vi "Rodriguez_Ex3Task1_Main.vi"() -> ()   [LabVIEW 2014, in "Rodriguez1_Visage_5th_LegoRobotics_11-29-16.lvrbt"]
uses:
  Rodriguez1_Visage_5th_LegoRobotics_11-29-16.lvrbt
panel:
  out "Current Distance":dbl
  in  "Max Distance":dbl
  in  "Min Distance":dbl
  out "Wall Proximity":string
  out "Distance LED":bool
  in  "stop":bool
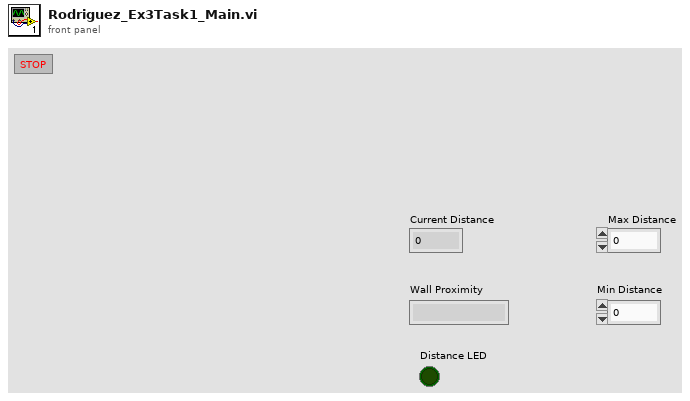
[diagram p1: front panel]
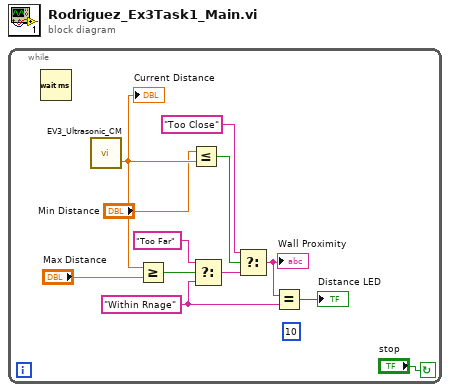
[diagram p0: block diagram]
diagram:
  n1 = while {
    stop <- "stop" continue-if-true
    (unwired) u32 10 ("millisecond timer value")
    w4 = "Within Rnage"
    n2 = Wait (ms)() -> ()  [unwired: 1 in, 1 out]
    n3 = call <vilib>:"EV3_Ultrasonic_CM.vi"() -> ("Centimeters"=w11:sgl)  [unwired: 3 in, 1 out]
    "Current Distance" <- w11
    n4 = Greater Or Equal?(x=w11, y="Max Distance") -> (x >= y?=w8:bool)
    n5 = Less Or Equal?(x="Min Distance", y=w11) -> (x <= y?=w9:bool)
    n6 = Select(t="Too Far", s=w8, f=w4) -> (s? t:f=w7:string)
    n7 = Select(t="Too Close", s=w9, f=w7) -> (s? t:f=w2:string)
    "Wall Proximity" <- w2
    n8 = Equal?(x=w2, y=w4) -> (x = y?=→"Distance LED":bool)
  }
